vi "SerialBusHound - 複製 (2).vi"() -> ()   [LabVIEW 2011]
uses:
  <vilib>/Platform/TimedLoop/XDataNode/timing_clust.ctl
  <vilib>/Platform/TimedLoop/XDataNode/nitl_modes.ctl
  <vilib>/Platform/TimedLoop/XDataNode/wakeup.ctl
  Enumerator/CmdType.ctl
  Variable/gSTOP.vi
  <vilib>/Platform/TimedLoop/XDataNode/XDataNode.xnode
  <vilib>/Platform/TimedLoop/XDataNode/XDNodeRunTimeDep.lvlib
panel:
  in  "parity":u16(ring) items=["None", "Odd", "Even", "Mark", "Space"]
  in  "data bits":u16(ring)=8 items=["5"=5, "6"=6, "7"=7, "8"=8]
  in  "stop bits":u16(ring)=10 items=["1.0"=10, "1.5"=15, "2.0"=20]
  out "Card Info":string="25469:57693"
  out "status":bool
  in  "baud rate":u32=9600
  in  "visa-rs232":refnum<visa-resource-name>="COM5"
  in  "run":bool
  # "Serial Settings"
  # "Com Port :"
  # "Status :"
  # "Parity :"
  # "Stop Bits :"
  # "Baud Rate :"
  # "Data Bits :"
  # "Card Information"
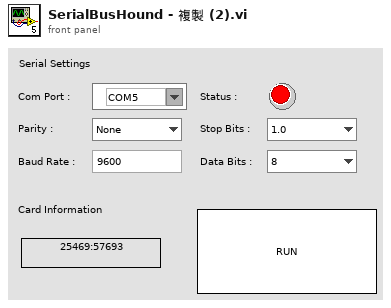
[diagram p1: front panel]
types:
  T1 = enum16{"Open", "R", "W", "R->W", "W->R", "Close"}
  T2 = enum16{"Obtain", "Enqueue", "Dequeue", "Release"}
  T3 = typedef "XDNodeRunTimeDep.lvlib/timing_clust.ctl" = cluster{"Expected End [f-1]":u64, "Actual End [f-1]":u64, "Finished Late? [f-1]":bool, "Expected End [i-1]":u64, "Actual End [i-1]":u64, "Finished Late? [i-1]":bool, "Expected Start [i]":u64, "Actual Start [i]":u64, "Expected Start [f]":u64, "Actual Start [f]":u64, "Source Name":string, "Structure Name":string, "Period":i64, "Deadline":i64, "Offset":i64, "Start":i64, "Priority":i32, "Timeout":i32, "Mode":T4, "Wakeup Reason":T5, "Error":errorcluster, "Source Type":string, "Secondary Source Type":string, "Global End Time":u64, "Global Start Time":u64, "Frame Duration":u64, "Iteration Duration":u64, "Assigned CPU":i32, "I/O Scan Engine Mode":u32}
  T4 = typedef "XDNodeRunTimeDep.lvlib/nitl_modes.ctl" = enum32{"No Change", "Process missed periods, maintain original phase", "Discard missed periods, maintain original phase", "Process missed periods, ignore original phase", "Discard missed periods, ignore original phase"}
  T5 = typedef "XDNodeRunTimeDep.lvlib/wakeup.ctl" = enum32{"Normal", "Aborted", "Asynchronous wakeup", "Timing source error", "Timed loop error", "Timeout"}
  T6 = typedef "CmdType.ctl" = enum16{"GetEventLog", "DelTransaction", "InvalidMessage", "RelayControl", "RelayOff", "RelayOn", "VaildMessage", "EventPolling", "StoppingWaiting", "PromptKeying-in"}
  T7 = cluster{"VISA-RS232":refnum<visa-resource-name>, "baud rate":u32, "data bits":u16, "parity":u16, "stop bits":u16}
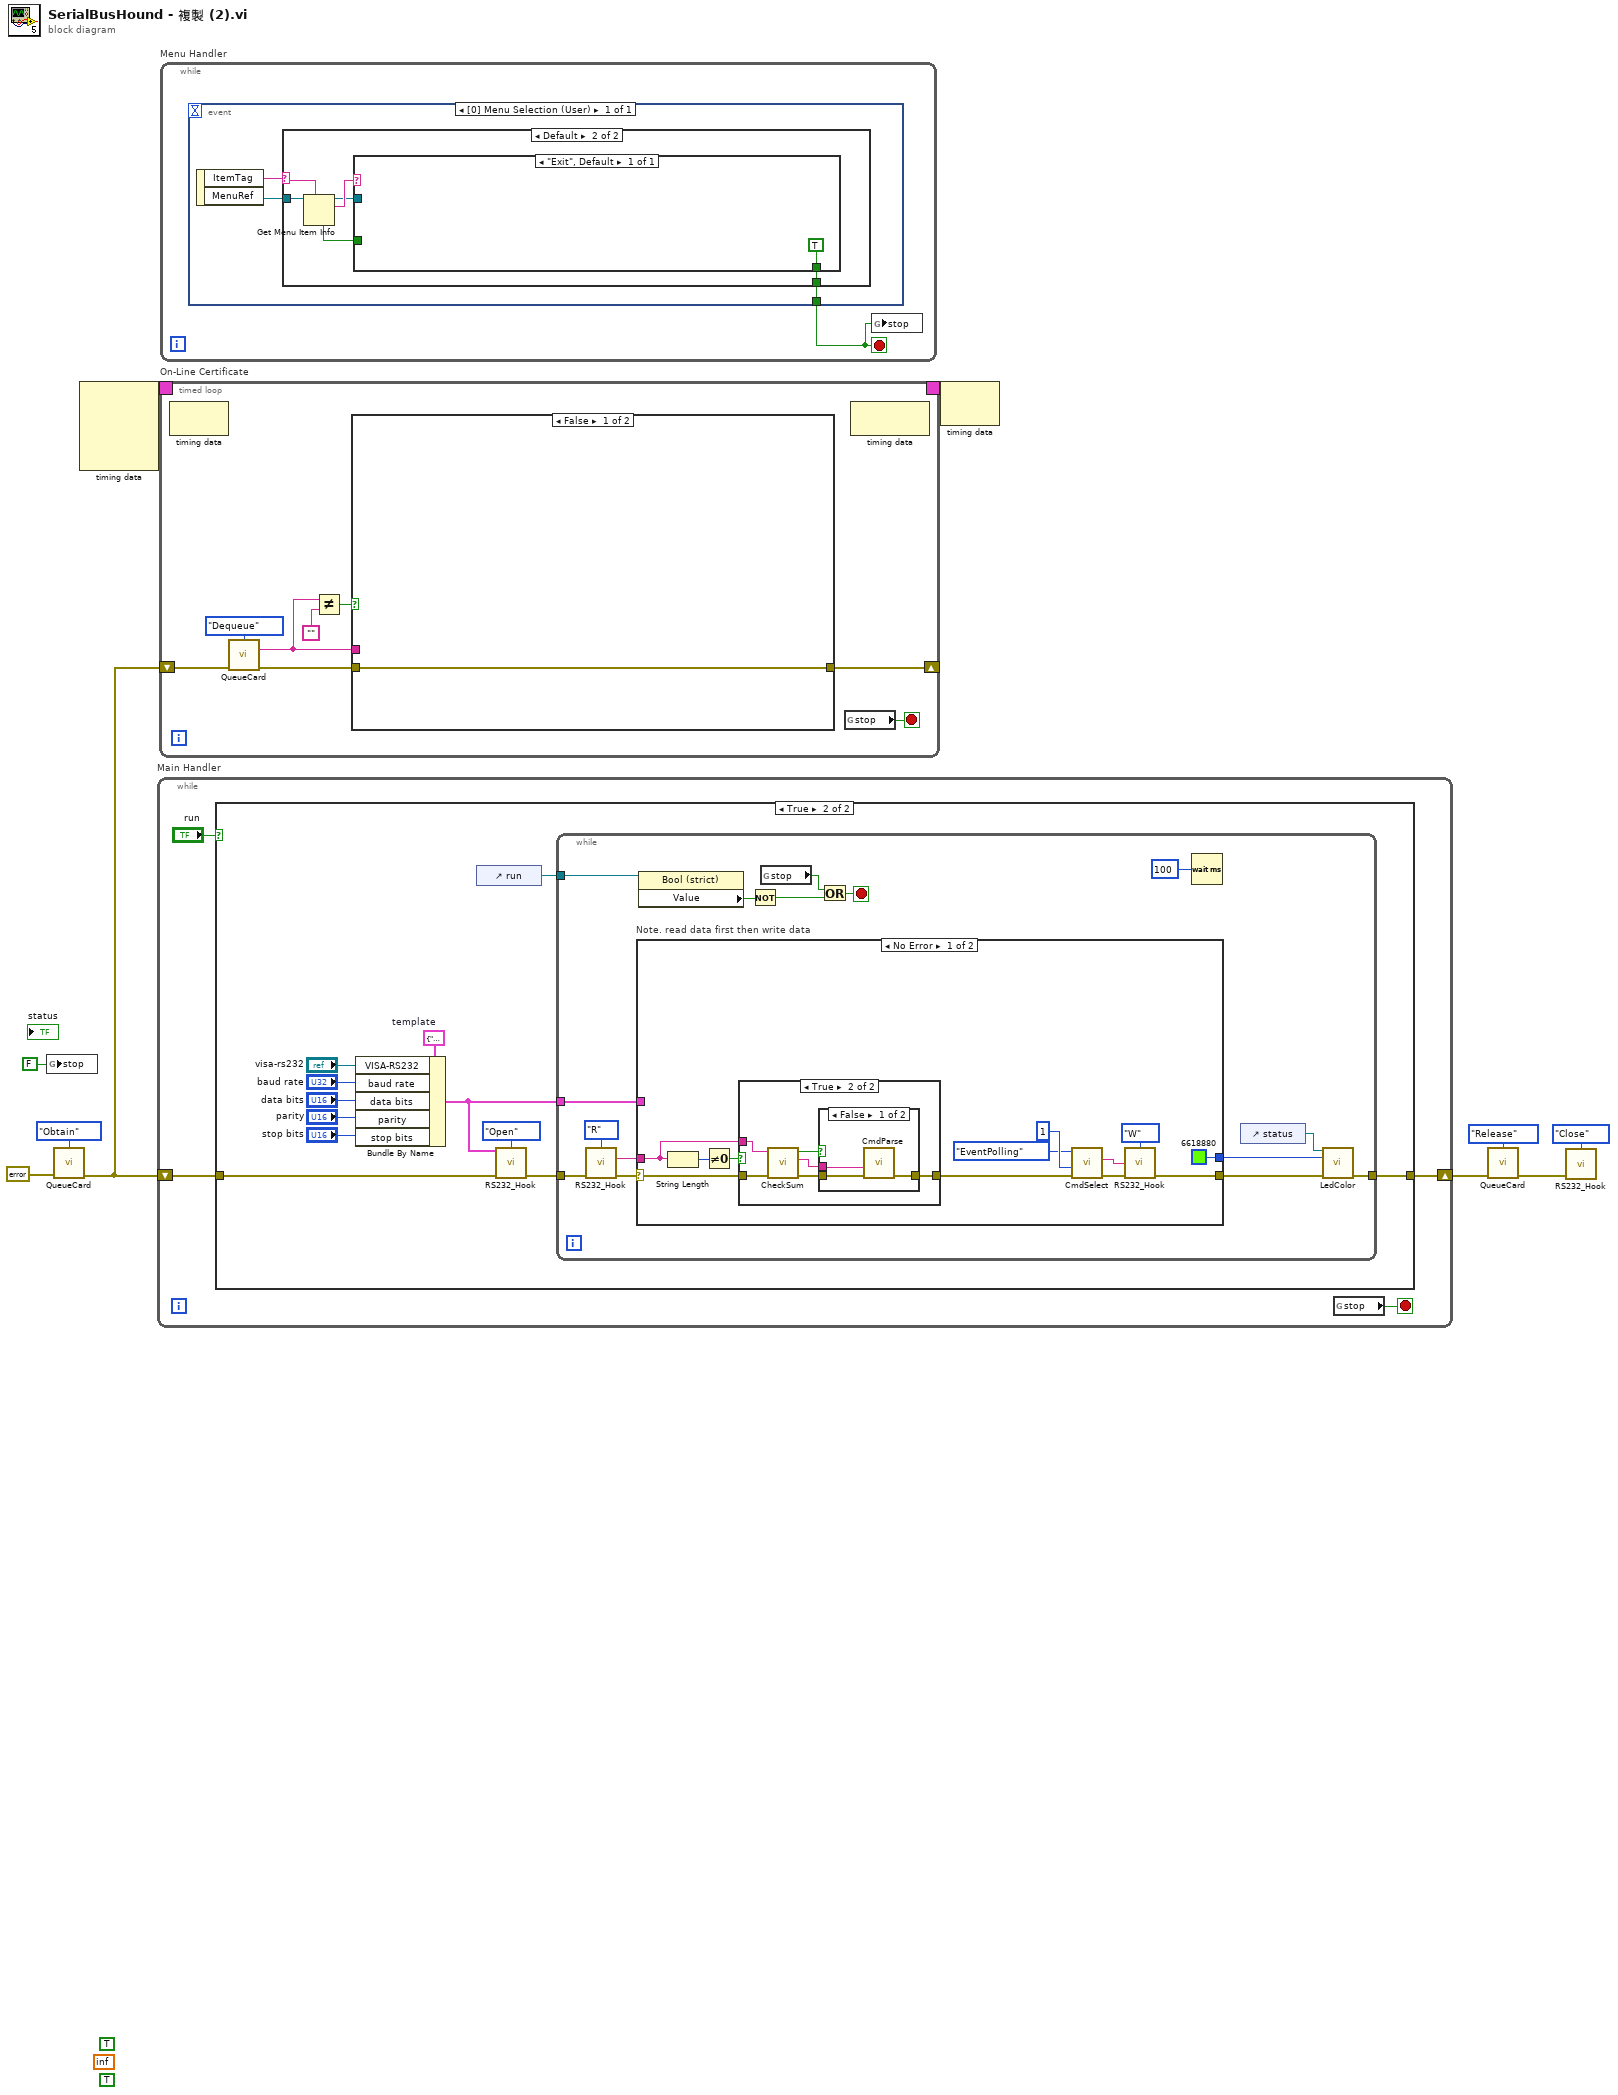
[diagram p0: block diagram]
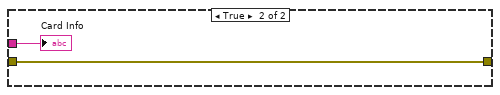
[diagram p2: hidden frame]
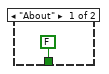
[diagram p3: hidden frame]
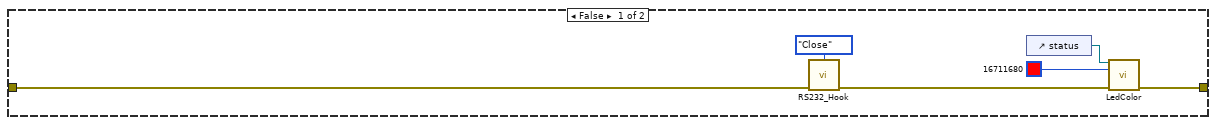
[diagram p4: hidden frame]
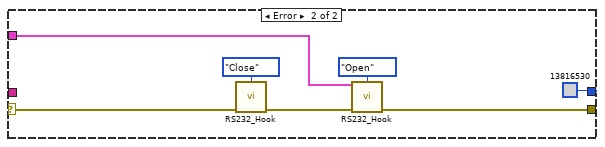
[diagram p7: hidden frame]
diagram:
  (unwired) TRUE ("Text.Font:Bold")
  (unwired) inf
  (unwired) TRUE ("Vertical Scrollbar Visible")
  n1 = global write "gSTOP.vi" "stop"(FALSE ("stop")) -> ()
  n2 = call "QueueCard.vi"("Mode"=T2."Obtain", "error in (no error)"=errorcluster {"status"=FALSE, "code"=0, "source"=""} ("error constant")) -> ("error out"=w5:errorcluster)  [unwired: 12 in, 1 out]
  n3 = node-c288() -> (w7:T3)  [unwired: 4 in]
  n4 = while "Main Handler" {
    shift-right: [w11] -> w8
    shift-left: w5 -> [w14]
    stop <- w13 stop-if-true
    n5 = case shown="True" "run" {
      tunnel: w14 -> [w19 w25]
      tunnel: [w16 w32] -> w11
      frame False {
        n6 = call "RS232_Hook.vi"("Mode"=T1."Close", "error in"=w19) -> ("error out"=w17:errorcluster)  [unwired: 12 in, 1 out]
        n7 = control-ref of="status"() -> (w18:refnum<vi>)
        n8 = call "LedColor.vi"("Boolean in"=w18, "Color Box"=u32 16711680, "error in (no error)"=w17) -> ("error out"=w16:errorcluster)  [unwired: 12 in]
      }
      frame True {
        w29 = T7 {"VISA-RS232"="", "baud rate"=0, "data bits"=0, "parity"=0, "stop bits"=0}  # template
        n9 = Bundle By Name(cluster=w29, "VISA-RS232"="visa-rs232", "baud rate"="baud rate", "data bits"="data bits", "parity"="parity", "stop bits"="stop bits") -> (w26:T7)
        n10 = control-ref of="run"() -> (w24:refnum<vi>)
        n11 = call "RS232_Hook.vi"("RS232 Config"=w26, "Mode"=T1."Open", "error in"=w25) -> ("error out"=w27:errorcluster)  [unwired: 11 in, 1 out]
        n12 = while {
          tunnel: [w33] -> w32
          tunnel: w27 -> [w47]
          tunnel: w26 -> [w46]
          tunnel: w24 -> [w41]
          stop <- w39 stop-if-true
          n13 = call "RS232_Hook.vi"("Mode"=T1."R", "error in"=w47) -> ("data out"=w44:string, "error out"=w45:errorcluster)  [unwired: 12 in]
          n14 = case "Note. read data first then write data" shown="No Error" w45 {
            selector: w45 -> [w50 w75]
            tunnel: [w48 w73] -> w34
            tunnel: w46 -> [_ w72]
            tunnel: w44 -> [w59 _]
            tunnel: [u32 6618880 u32 13816530] -> w35
            frame No Error {
              n15 = String Length(string=w59) -> (length=w52:i32)
              n16 = Not Equal To 0?(x=w52) -> (x != 0?=w51:bool)
              n17 = case shown="True" w51 {
                tunnel: w59 -> [_ w61]
                tunnel: w50 -> [w60 w63]
                tunnel: [w60 w62] -> w49
                frame False {
                }
                frame True {
                  n18 = call "CheckSum.vi"("error in (no error)"=w63, "string in"=w61) -> ("error out"=w64:errorcluster, "string out"=w66:string, "No Parse"=w65:bool)  [unwired: 7 in]
                  n19 = case shown="False" w65 {
                    tunnel: w64 -> [w69 w70]
                    tunnel: [w68 w70] -> w62
                    tunnel: w66 -> [w67 _]
                    frame False {
                      n20 = call "CmdParse.vi"("error in (no error)"=w69, "Read Buffer"=w67) -> ("error out"=w68:errorcluster)  [unwired: 9 in]
                    }
                    frame True {
                    }
                  }
                }
              }
              n21 = call "CmdSelect.vi"("error in (no error)"=w49, "Node Id"=u8 1, "Cmd Type"=CmdType."EventPolling") -> ("error out"=w57:errorcluster, "Cmd Str"=w53:string)  [unwired: 7 in]
              n22 = call "RS232_Hook.vi"("Mode"=T1."W", "data in"=w53, "error in"=w57) -> ("error out"=w48:errorcluster)  [unwired: 11 in, 1 out]
            }
            frame Error {
              n23 = call "RS232_Hook.vi"("Mode"=T1."Close", "error in"=w75) -> ("error out"=w74:errorcluster)  [unwired: 12 in, 1 out]
              n24 = call "RS232_Hook.vi"("RS232 Config"=w72, "Mode"=T1."Open", "error in"=w74) -> ("error out"=w73:errorcluster)  [unwired: 11 in, 1 out]
            }
          }
          n25 = property class="Bool (strict)"(reference=w41) -> ("Value"=w40:bool)  [unwired: 1 in, 2 out]
          n26 = Not(x=w40) -> (.not. x?=w37:bool)
          n27 = global read "gSTOP.vi" "stop"() -> (w38:bool)
          n28 = Or(x=w38, y=w37) -> (x .or. y?=w39:bool)
          n29 = Wait (ms)(milliseconds to wait=u32 100 ("ms")) -> ()  [unwired: 1 out]
          n30 = control-ref of="status"() -> (w36:refnum<vi>)
          n31 = call "LedColor.vi"("Boolean in"=w36, "Color Box"=w35, "error in (no error)"=w34) -> ("error out"=w33:errorcluster)  [unwired: 12 in]
        }
      }
    }
    n32 = global read "gSTOP.vi" "stop"() -> (w13:bool)
  }
  n33 = timed-loop "On-Line Certificate" {
    shift-right: [w81] -> _
    shift-left: w5 -> [w84]
    timing: w7 -> [_]
    timing-out: [_] -> w6
    stop <- w79 stop-if-true
    n34 = node-c288() -> ()  [unwired: 1 in, 1 out]
    n35 = call "QueueCard.vi"("Mode"=T2."Dequeue", "error in (no error)"=w84) -> ("Queue Out"=w78:string, "error out"=w82:errorcluster)  [unwired: 12 in]
    n36 = Not Equal?(x=w78, y="") -> (x != y?=w83:bool)
    n37 = case shown="False" w83 {
      tunnel: w82 -> [w88 w90]
      tunnel: [w88 w90] -> w81
      tunnel: w78 -> [_ w89]
      frame False {
      }
      frame True {
        "Card Info" <- w89
      }
    }
    n38 = global read "gSTOP.vi" "stop"() -> (w79:bool)
    n39 = node-c288() -> ()  [unwired: 1 in, 1 out]
  }
  n40 = while "Menu Handler" {
    stop <- w91 stop-if-true
    n41 = event shown="[0] Menu Selection (User)" {
      selector: _ -> [_]
      dyn-events: _ -> [_]
      timeout: _ -> [_]
      tunnel: [w92] -> w91
      event Menu Selection (User) {
        n42 = event-data() -> ("ItemTag"=w93:string, "MenuRef"=w94:refnum<k9>)  [unwired: 1 in]
        n43 = case shown="Default" w93 {
          selector: w93 -> [_ w100]
          tunnel: w94 -> [_ w101]
          tunnel: [FALSE w98] -> w92
          frame "About" {
          }
          frame Default {
            n44 = Get Menu Item Info(7:w100, 11:w101) -> (2:w99:string, 3:w97:refnum<k9>, 4:w96:bool)  [unwired: 1 in, 4 out]
            n45 = case shown="\"Exit\", Default" w99 {
              tunnel: [TRUE] -> w98
              tunnel: w97 -> [_]
              tunnel: w96 -> [_]
              frame "Exit", Default {
              }
            }
          }
        }
      }
    }
    n46 = global write "gSTOP.vi" "stop"(w91) -> ()
  }
  n47 = node-c288(w6) -> ()  [unwired: 1 out]
  n48 = call "QueueCard.vi"("Mode"=T2."Release", "error in (no error)"=w8) -> ("error out"=w1:errorcluster)  [unwired: 12 in, 1 out]
  n49 = call "RS232_Hook.vi"("Mode"=T1."Close", "error in"=w1) -> ()  [unwired: 12 in, 2 out]
